vi "REPORT_CFG_filter_records.vi"(9 "REPORT_CFG_filters":T1={"order_selection"=enum."new_to_old", "OP"=""}, 11 "records":string[][](array[string])) -> (3 "ItemNames":string[][](array[string]))   [LabVIEW 2019]
uses:
  typedef/REPORT_CFG_filters.ctl
  <userlib>/_OpenG.lib/array/array.llb/Reverse 2D Array (String)__ogtk.vi
  <userlib>/_OpenG.lib/array/array.llb/Filter 1D Array with Scalar (String)__ogtk.vi
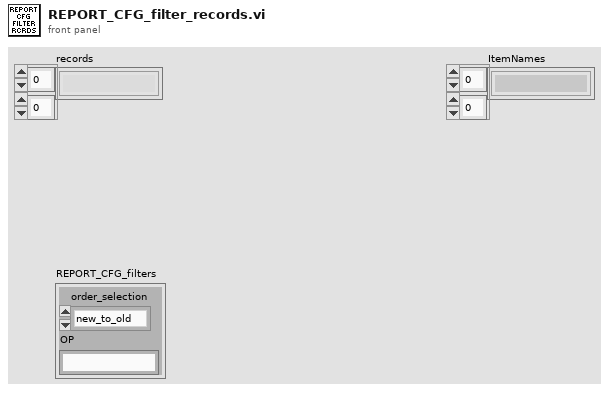
[diagram p1: front panel]
types:
  T1 = typedef "REPORT_CFG_filters.ctl" = cluster{"order_selection":enum32{"old_to_new", "new_to_old"}, "OP":string}
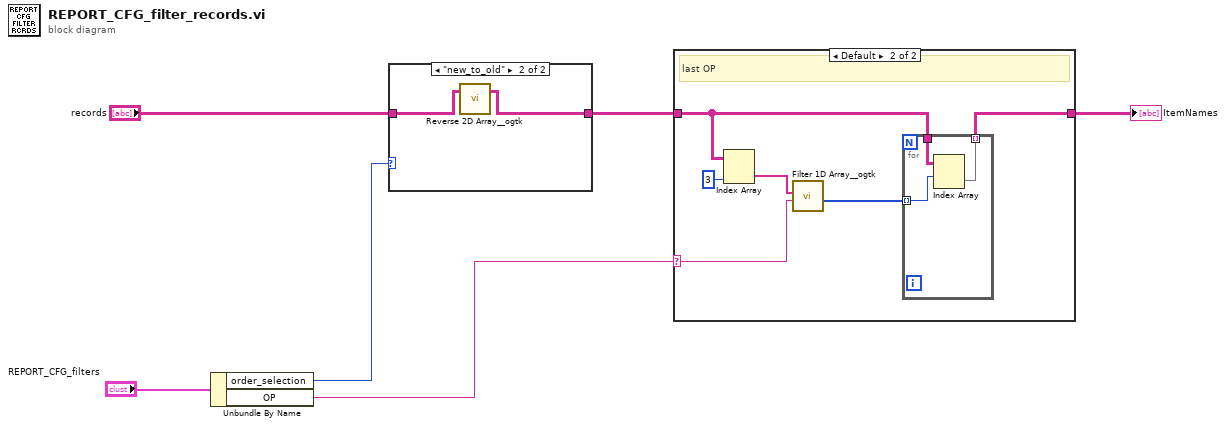
[diagram p0: block diagram]
diagram:
  n1 = Unbundle By Name("REPORT_CFG_filters") -> ("order_selection"=w4:enum32{"old_to_new", "new_to_old"}, "OP"=w3:string)
  n2 = case shown="\"new_to_old\"" w4 {
    tunnel: "records" -> [w7 w9]
    tunnel: [w7 w8] -> w2
    frame "old_to_new" {
    }
    frame "new_to_old" {
      n3 = call-poly <userlib>:"Reverse 2D Array__ogtk.vi"("Array"=w9) -> ("Reversed Array"=w8:string[][])  [unwired: 2 in]
    }
  }
  n4 = case shown="Default" w3 {
    selector: w3 -> [_ w16]
    tunnel: [w10 w13] -> w1
    tunnel: w2 -> [w10 w11]
    frame "ALL" {
      # "OP"
    }
    frame Default {
      # "last OP"
      n5 = Index Array(array=w11, index (col)=3 ("disabled index (col)")) -> (element=w14:string[])  [unwired: 1 in]
      n6 = call-poly <userlib>:"Filter 1D Array__ogtk.vi"("items to filter"=w16, "array"=w14) -> ("filtered item indices"=w12:i32[])  [unwired: 4 in, 1 out]
      n7 = for {
        tunnel: w11 -> [w19]
        tunnel: w12 -> [w17] mode=indexing
        tunnel: [w18] -> w13 mode=indexing
        n8 = Index Array(array=w19, index (row)=w17) -> (element=w18:string[])  [unwired: 1 in]
      }
    }
  }
  "ItemNames" <- w1
